vi "DataTypes.vi"() -> ()   [LabVIEW 2019]
panel:
  out "Indvar3":string
  out "Indvar2":u8
  out "Indvar1":dbl
  in  "var3":string
  in  "var2":u8
  in  "var1":dbl
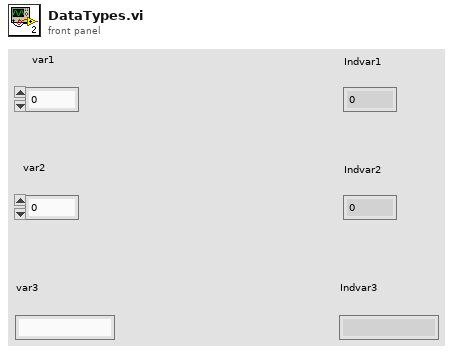
[diagram p1: front panel]
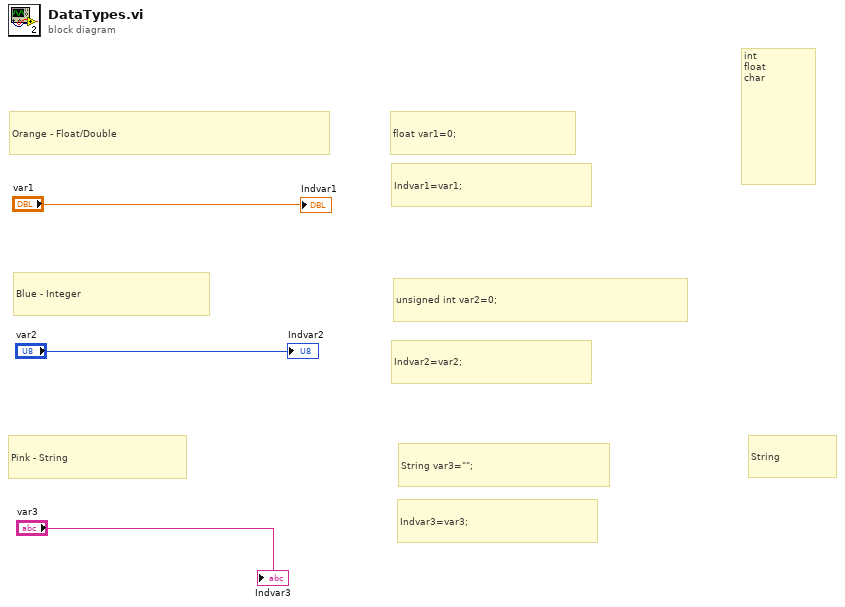
[diagram p0: block diagram]
diagram:
  # "Indvar3=var3;"
  # "Indvar2=var2;"
  # "Indvar1=var1;"
  # "String var3=\"\";"
  # "Pink - String"
  # "String"
  # "Blue - Integer"
  # "unsigned int var2=0;"
  # "float var1=0;"
  # "Orange - Float/Double"
  # "int\nfloat\nchar"
  "Indvar1" <- "var1"
  "Indvar2" <- "var2"
  "Indvar3" <- "var3"
